vi "dfd_CIC_IntegratorStage.vi"(10 "input valid":bool, 11 "data in":bool[](array[boolean])) -> (2 "output valid":bool, 3 "data out":bool[](array[boolean]))   [LabVIEW 2017]
uses:
  <vilib>/rvi/FXPMathLib/basic elements/FxpIntAccumulator/simVIs/DllFxpIntAccumulator_sub.vi
  <vilib>/rvi/FXPMathLib/basic elements/FxpDiscreteDelay/XNode/nifxpmath_DiscreteDelay.xnode
  <vilib>/rvi/FXPMathLib/basic elements/FxpIntAccumulator/XNode/nifxpmath_IntAccumulator.xnode
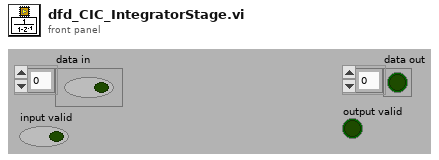
[diagram p1: front panel]
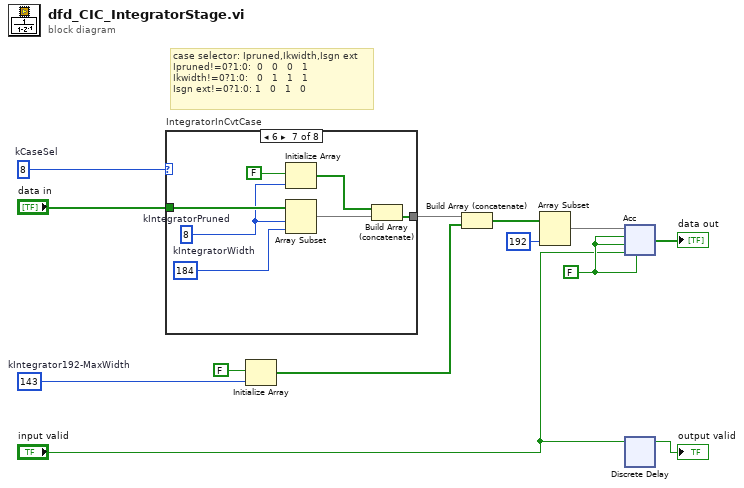
[diagram p0: block diagram]
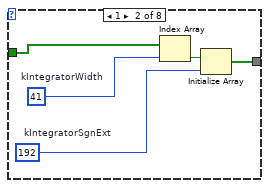
[diagram p3: hidden frame]
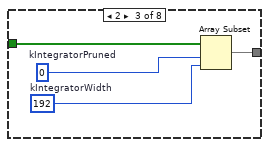
[diagram p4: hidden frame]
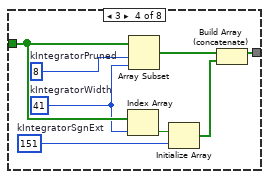
[diagram p5: hidden frame]
diagram:
  w11 = FALSE ("load")
  w8 = 143  # kIntegrator192-MaxWidth
  w3 = 8  # kCaseSel
  # "case selector: Ipruned,Ikwidth,Isgn ext\nIpruned!=0?1:0:  0   0   0   1\nIkwidth!=0?1:0:   0   1   1   1\nIsgn ext!=0?1:0: 1   0   1   0"
  n1 = case "IntegratorInCvtCase" shown="6" w3 {
    tunnel: "data in" -> [w14 w19 w23 w31 w32 w33 w40 w41]
    tunnel: [w14 w17 w22 w27 w32 w33 w36 w41] -> w6
    frame 0, Default {
    }
    frame 1 {
      w15 = 192  # kIntegratorSgnExt
      w16 = 41  # kIntegratorWidth
      n2 = Index Array(array=w19, index=w16) -> (element=w18:bool)
      n3 = Initialize Array(w18, w15) -> (w17:bool[])
    }
    frame 2 {
      w20 = 192  # kIntegratorWidth
      w21 = 0  # kIntegratorPruned
      n4 = Array Subset(array=w23, index=w21, length=w20) -> (w22:bool[])
    }
    frame 3 {
      w24 = 151  # kIntegratorSgnExt
      w25 = 41  # kIntegratorWidth
      w26 = 8  # kIntegratorPruned
      n5 = Index Array(array=w31, index=w25) -> (element=w28:bool)
      n6 = Array Subset(array=w31, index=w26, length=w25) -> (w30:bool[])
      n7 = Initialize Array(w28, w24) -> (w29:bool[])
      n8 = Build Array (concatenate)(w30, w29) -> (w27:bool[])
    }
    frame 4 {
    }
    frame 5 {
    }
    frame 6 {
      w34 = 184  # kIntegratorWidth
      w35 = 8  # kIntegratorPruned
      n9 = Initialize Array(FALSE, w35) -> (w37:bool[])
      n10 = Array Subset(array=w40, index=w35, length=w34) -> (w39:bool[])
      n11 = Build Array (concatenate)(w37, w39) -> (w36:bool[])
    }
    frame 7 {
    }
  }
  n12 = Initialize Array(FALSE, w8) -> (w5:bool[])
  n13 = Build Array (concatenate)(w6, w5) -> (w4:bool[])
  n14 = Array Subset(array=w4, length=192) -> (w2:bool[])  [unwired: 1 in]
  n15 = xnode ("Acc")("x"=w2, "load (F)"=w11, "is sub? (F)"=w11, "enable (T)"="input valid", "carry-in/inverted borrow-in (F)"=w11) -> ("s"=→"data out":bool[])  [unwired: 1 out]
  n16 = xnode ("Discrete Delay")("D"="input valid") -> ("Q"=→"output valid":bool)
